vi "Load PNG Image.vi"(8 "error in (no error)":errorcluster, 11 "Picture in":path) -> (0 "error out":errorcluster, 3 "Image out":refnum<class "Image.lvclass">)   [LabVIEW 2021, in "Menu.lvlib" / "Menu.lvclass"]
uses:
  Menu.lvclass
  Menu.lvclass/Menu.ctl
  Picture2D/src/Picture/Image.lvclass
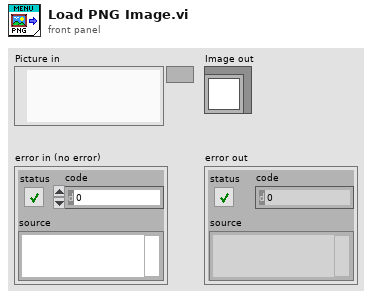
[diagram p1: front panel]
types:
  T1 = typedef "imagedata.ctl" = cluster{"image type":i32, "image depth":i32, "image":u8[], "mask":u8[], "colors":u32[], "Rectangle":cluster{"left":i16, "top":i16, "right":i16, "bottom":i16}}
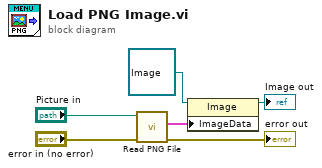
[diagram p0: block diagram]
diagram:
  n1 = call <vilib>:"Read PNG File.vi"("error in (no error)"="error in (no error)", "path to PNG file"="Picture in") -> ("error out"=→"error out":errorcluster, "image data"=w4:T1)  [unwired: 7 in, 1 out]
  n2 = property class="Image"(reference=refnum<class "Image.lvclass"> refnum ("Picture"), "ImageData"=w4) -> (reference out=→"Image out":refnum<class "Image.lvclass">)  [unwired: 1 in, 1 out]
